vi "SCTopLevel.vi"   [LabVIEW 2014]
uses:
  Controls/SPstate.ctl
  <vilib>/Platform/TimedLoop/XDataNode/timing_clust.ctl
  <vilib>/Platform/TimedLoop/XDataNode/nitl_modes.ctl
  <vilib>/Platform/TimedLoop/XDataNode/wakeup.ctl
  <vilib>/rvi/Emulation/niFpgaGetClockAttributes.vi
  <vilib>/rvi/Emulation/niFpgaSctlEmulationGetInTimedLoop.vi
  <vilib>/rvi/Emulation/niFpgaEmulationReportErrorSimple.vi
  <vilib>/rvi/Emulation/niFpgaCriticalErrorInLSC.vi
  <vilib>/rvi/Emulation/niFpgaEmulationIsFPGAContextNoSignature.vi
  <vilib>/rvi/DataTransferAndStorage/Container/Common/niFpgaContainerGetUniqueNameForEmu.vi
  <vilib>/rvi/eio/common/nirviEmuReportErrorAndStop.vi
  <vilib>/rvi/Emulation/niFpgaProcessEmulError.vi
  SCGlobVars.vi
  <vilib>/Platform/TimedLoop/XDataNode/XDataNode.xnode
  <vilib>/rvi/DataTransferAndStorage/Container/XNode/niFpgaContainer.xnode
  <vilib>/rvi/DataTransferAndStorage/Handshake/Emulation/niFpgaHandshakeEmulation.vi
  <vilib>/Platform/TimedLoop/XDataNode/XDNodeRunTimeDep.lvlib
types:
  T1 = typedef "SPstate.ctl" = enum16{"idle", "scanning", "done", "error"}
  T2 = typedef "XDNodeRunTimeDep.lvlib/timing_clust.ctl" = cluster{"Expected End [f-1]":u64, "Actual End [f-1]":u64, "Finished Late? [f-1]":bool, "Expected End [i-1]":u64, "Actual End [i-1]":u64, "Finished Late? [i-1]":bool, "Expected Start [i]":u64, "Actual Start [i]":u64, "Expected Start [f]":u64, "Actual Start [f]":u64, "Source Name":string, "Structure Name":string, "Period":i64, "Deadline":i64, "Offset":i64, "Start":i64, "Priority":i32, "Timeout":i32, "Mode":T3, "Wakeup Reason":T4, "Error":errorcluster, "Source Type":string, "Secondary Source Type":string, "Global End Time":u64, "Global Start Time":u64, "Frame Duration":u64, "Iteration Duration":u64, "Assigned CPU":i32, "I/O Scan Engine Mode":u32}
  T3 = typedef "XDNodeRunTimeDep.lvlib/nitl_modes.ctl" = enum32{"No Change", "Process missed periods, maintain original phase", "Discard missed periods, maintain original phase", "Process missed periods, ignore original phase", "Discard missed periods, ignore original phase"}
  T4 = typedef "XDNodeRunTimeDep.lvlib/wakeup.ctl" = enum32{"Normal", "Aborted", "Asynchronous wakeup", "Timing source error", "Timed loop error", "Timeout"}
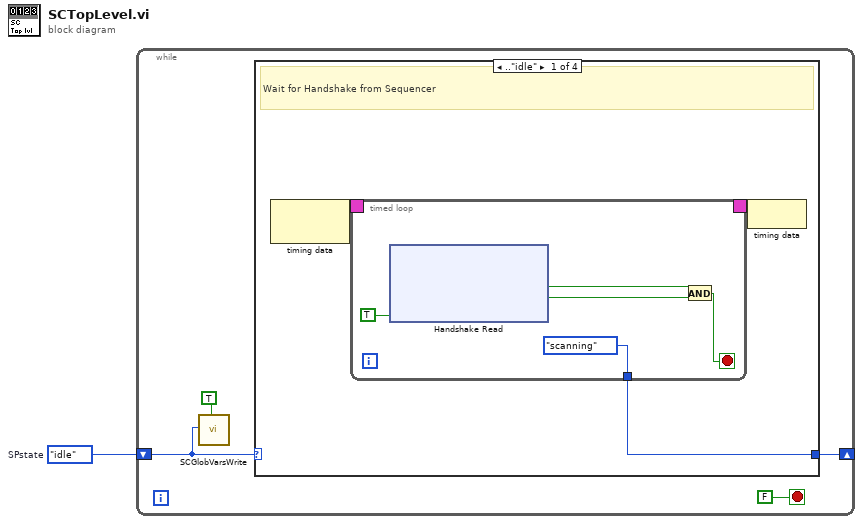
[diagram p0: block diagram]
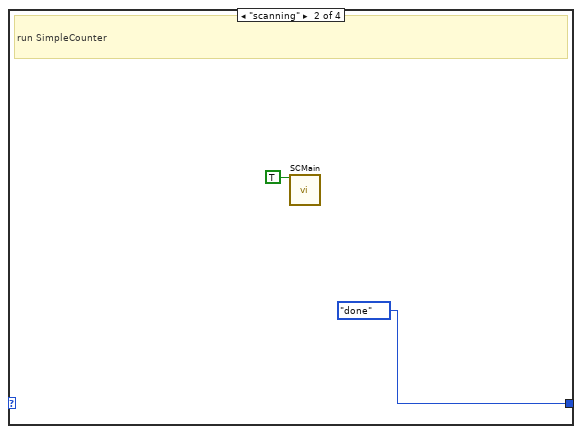
[diagram p2: hidden frame]
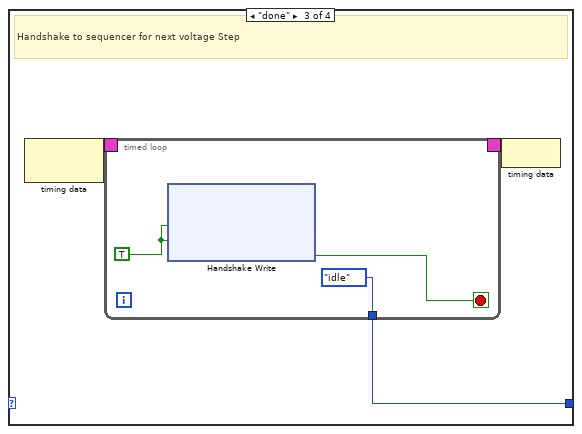
[diagram p3: hidden frame]
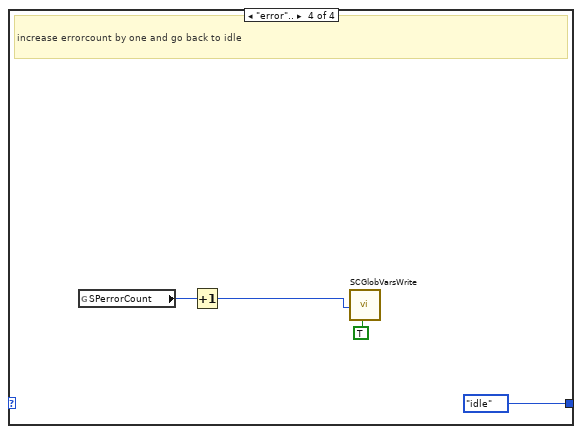
[diagram p4: hidden frame]
diagram:
  w1 = SPstate."idle"  # SPstate
  n1 = while {
    shift-right: [w4] -> _
    shift-left: w1 -> [w3]
    stop <- FALSE stop-if-true
    n2 = call "SCGlobVarsWrite.vi"("SPstate"=w3, "writeStateOnly"=TRUE) -> ()  [unwired: 18 in]
    n3 = case shown="..\"idle\"" w3 {
      tunnel: [w6 SPstate."done" ("SPstate") w20 SPstate."idle" ("SPstate")] -> w4
      frame .."idle" {
        # "Wait for Handshake from Sequencer"
        n4 = node-c288() -> (w8:T2)  [unwired: 1 in]
        n5 = timed-loop {
          timing: w8 -> [_]
          timing-out: [_] -> w7
          tunnel: [SPstate."scanning" ("SPstate")] -> w6
          stop <- w10 stop-if-true
          n6 = xnode ("Handshake Read")("Ready for Output"=TRUE) -> ("Data"=w12:bool, "Output Valid"=w11:bool)  [unwired: 1 in, 1 out]
          n7 = And(x=w12, y=w11) -> (x .and. y?=w10:bool)
        }
        n8 = node-c288(w7) -> ()
      }
      frame "scanning" {
        # "run SimpleCounter"
        n9 = call "SCMain.vi"("once?"=TRUE) -> ()  [unwired: 19 in]
      }
      frame "done" {
        # "Handshake to sequencer for next voltage Step"
        n10 = node-c288() -> (w22:T2)  [unwired: 1 in]
        n11 = timed-loop {
          timing: w22 -> [_]
          timing-out: [_] -> w21
          tunnel: [SPstate."idle" ("SPstate")] -> w20
          stop <- w25 stop-if-true
          w24 = TRUE ("Ready for Output")
          n12 = xnode ("Handshake Write")("Data"=w24, "Input Valid"=w24) -> ("Ready for Input"=w25:bool)  [unwired: 1 in, 1 out]
        }
        n13 = node-c288(w21) -> ()
      }
      frame "error".. {
        # "increase errorcount by one and go back to idle"
        n14 = global read "SCGlobVars.vi" "SPerrorCount"() -> (w30:u8)
        n15 = Increment(x=w30) -> (x+1=w31:u8)
        n16 = call "SCGlobVarsWrite.vi"("SPerrorCount"=w31, "writeErrorCountOnly"=TRUE ("writeOnlyErrorCount")) -> ()  [unwired: 18 in]
      }
    }
  }
